vi "Check if Valid and Generate Error.vi"(5 "generate error if invalid (F)":bool, 7 "chain levels to remove (2)":i32=2, 8 "error in (no error)":errorcluster, 11 "sentence":string) -> (0 "error out":errorcluster, 3 "valid sentence":bool)   [LabVIEW 2017, in "NMEA API.lvlib"]
uses:
  <vilib>/robotics/Protocols/NMEA/NMEA API.lvlib
  <vilib>/robotics/Utilities/NI_Robotics Utilities.lvlib
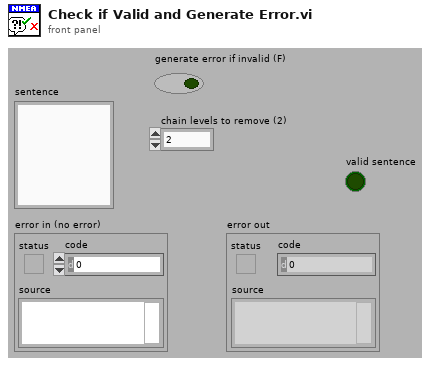
[diagram p1: front panel]
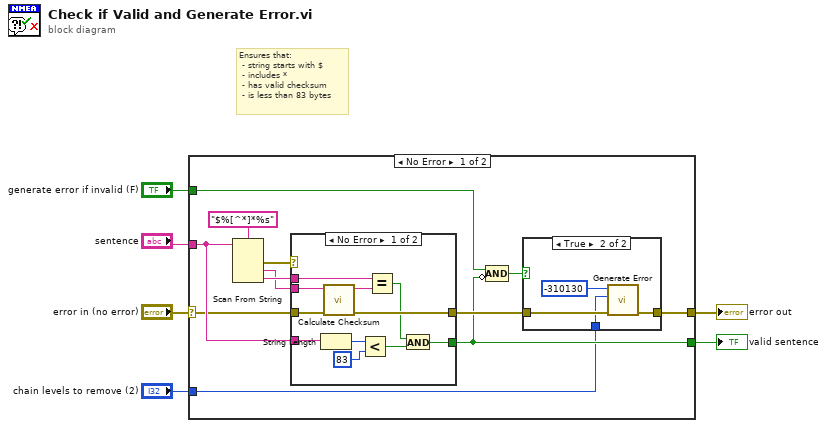
[diagram p0: block diagram]
diagram:
  # "Ensures that: \n - string starts with $ \n - includes * \n - has valid checksum\n - is less than 83 bytes"
  n1 = case shown="No Error" "error in (no error)" {
    selector: "error in (no error)" -> [w13 w36]
    tunnel: "sentence" -> [w16 _]
    tunnel: [w8 w36] -> w3
    tunnel: [w10 _] -> w4
    tunnel: "generate error if invalid (F)" -> [w11 _]
    tunnel: "chain levels to remove (2)" -> [w7 _]
    frame No Error {
      n2 = Scan From String(format string="$%[^*]*%s", input string=w16) -> (error out=w14:errorcluster, output 1=w15:string, output 2=w17:string)  [unwired: 2 in, 4 out]
      n3 = case shown="No Error" w14 {
        tunnel: w17 -> [w34 _]
        tunnel: w16 -> [w33 _]
        tunnel: [w24 _] -> w10
        tunnel: w15 -> [w30 _]
        tunnel: [w28 w35] -> w12
        tunnel: w13 -> [w27 w35]
        frame No Error {
          n4 = String Length(string=w33) -> (length=w32:i32)
          n5 = call <vilib>:"Calculate Checksum.vi"("error in (no error)"=w27, "string"=w30) -> ("error out"=w28:errorcluster, "checksum"=w29:string)  [unwired: 6 in]
          n6 = Less?(x=w32, y=83) -> (x < y?=w26:bool)
          n7 = Equal?(x=w34, y=w29) -> (x = y?=w25:bool)
          n8 = And(x=w25, y=w26) -> (x .and. y?=w24:bool)
        }
        frame Error {
        }
      }
      n9 = Compound Arithmetic op=AND(w11, invert w10) -> (w9:bool)
      n10 = case shown="True" w9 {
        tunnel: w12 -> [w19 w23]
        tunnel: [w19 w22] -> w8
        tunnel: w7 -> [_ w20]
        frame False {
        }
        frame True {
          n11 = call <vilib>:"Generate Error.vi"("error in (no error)"=w23, "chain levels to remove (1)"=w20, "code"=-310130) -> ("error out"=w22:errorcluster)  [unwired: 8 in]
        }
      }
    }
    frame Error {
    }
  }
  "valid sentence" <- w4
  "error out" <- w3
